vi "correlation_subVI.vi"(0 "signal":dbl[](array[numeric]), 1 "compare":dbl[](array[numeric])) -> (3 "max index":i32, 4 "max value":dbl, 5 "correlation":cluster{i32, i32, dbl[]}(graph))   [LabVIEW 2014]
uses:
  <vilib>/Analysis/2dsp.llb/1D Cross Correlation (DBL).vi
  <vilib>/Analysis/NI_AALPro.lvlib
panel:
  in  "stop":bool
  out "compare_size":i32
  out "signal_size":i32
  out "byCorrelationVI":cluster{i32, i32, "Rxy":dbl[]}(graph)
  out "compare_graph":dbl[](graph)
  out "signal_graph":dbl[](graph)
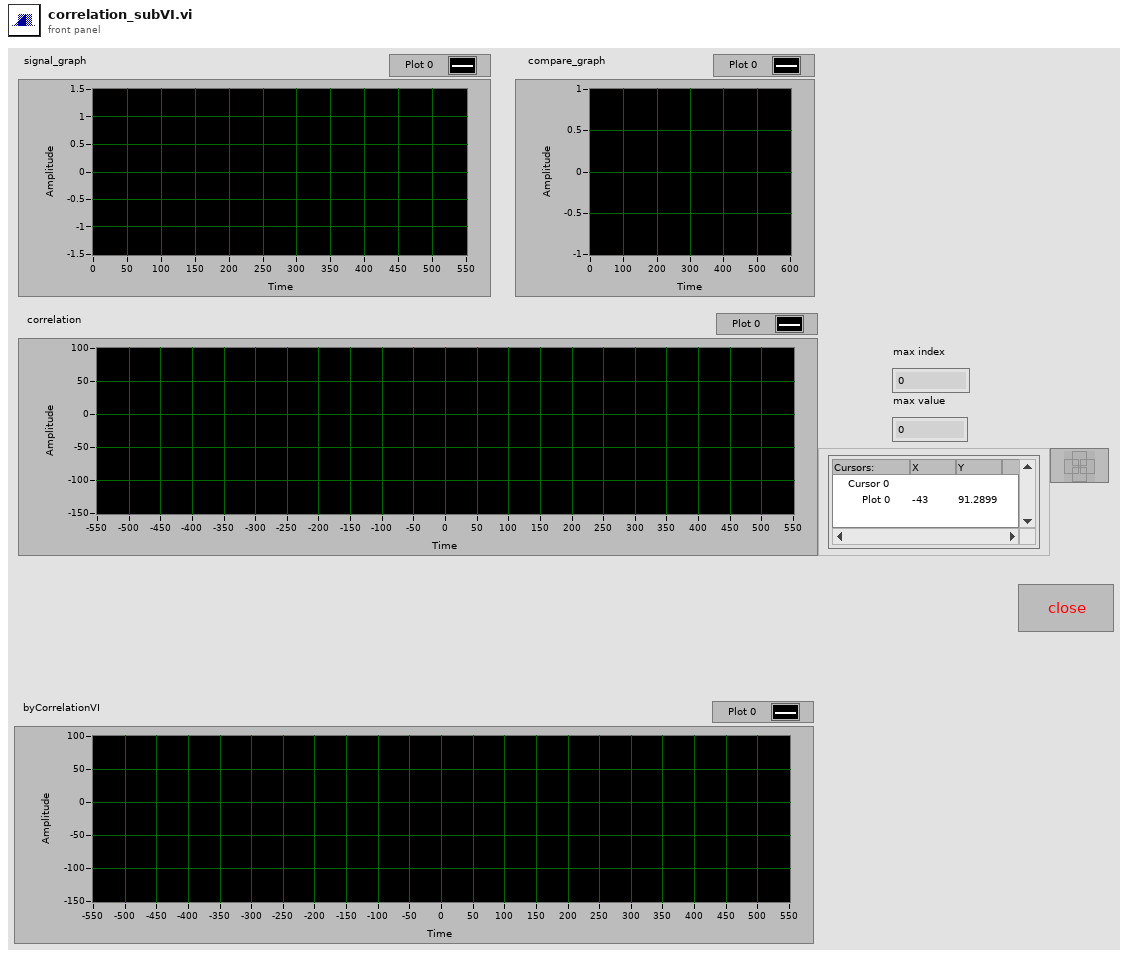
[diagram p1: front panel]
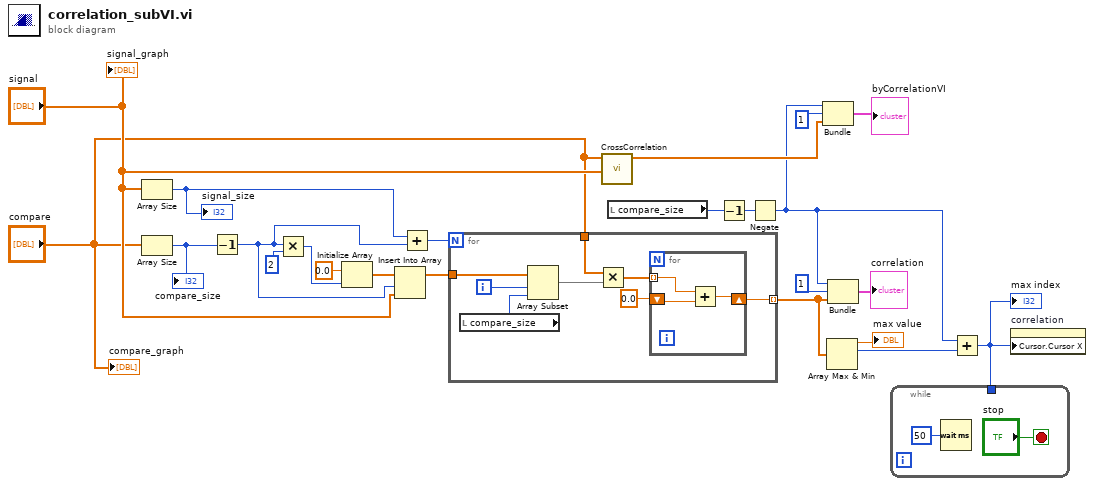
[diagram p0: block diagram]
diagram:
  n1 = Array Size(array="signal") -> (size(s)=w6:i32)
  "signal_size" <- w6
  n2 = Array Size(array="compare") -> (size(s)=w7:i32)
  "compare_size" <- w7
  n3 = Decrement(x=w7) -> (x-1=w3:i32)
  n4 = Multiply(x=w3, y=2) -> (x*y=w19:i32)
  n5 = Initialize Array(0.0 ("element"), w19) -> (w18:dbl[])
  n6 = Insert Into Array(array=w18, index=w3, new element="signal") -> (w17:dbl[])
  n7 = Add(x=w6, y=w3) -> (x+y=w22:i32)
  n8 = for {
    N: w22 -> [_]
    tunnel: [w24] -> w13 mode=indexing
    tunnel: "compare" -> [w27]
    tunnel: w17 -> [w26]
    i -> [w30]
    n9 = local read "compare_size"() -> (w25:i32)
    n10 = Array Subset(array=w26, index=w30, length=w25) -> (w28:dbl[])
    n11 = Multiply(x=w27, y=w28) -> (x*y=w31:dbl[])
    n12 = for {
      tunnel: w31 -> [w34] mode=indexing
      shift-right: [w33] -> w24
      shift-left: 0.0 -> [w32]
      n13 = Add(x=w34, y=w32) -> (x+y=w33:dbl)
    }
  }
  n14 = call-poly <vilib>:"CrossCorrelation.vi"("Y"="signal", "X"="compare") -> ("Rxy"=w11:dbl[])  [unwired: 8 in, 1 out]
  n15 = local read "compare_size"() -> (w5:i32)
  n16 = Decrement(x=w5) -> (x-1=w4:i32)
  n17 = Negate(x=w4) -> (-x=w10:i32)
  n18 = Bundle(w10, 1, "Rxy"=w11) -> (→"byCorrelationVI":cluster{i32, i32, "Rxy":dbl[]})  [unwired: 1 in]
  n19 = Array Max & Min(array=w13) -> (max value=→"max value":dbl, max index (indices)=w15:i32)  [unwired: 2 out]
  n20 = Bundle(w10, 1, w13) -> (→"correlation":cluster{i32, i32, dbl[]})  [unwired: 1 in]
  n21 = Add(x=w10, y=w15) -> (x+y=w12:i32)
  "max index" <- w12
  n22 = while {
    tunnel: w12 -> [_]
    stop <- "stop" stop-if-true
    n23 = Wait (ms)(milliseconds to wait=u32 50) -> ()  [unwired: 1 out]
  }
  n24 = property on="correlation" class="WFGraph (strict)"("Cursor.Cursor X"=w12) -> ()  [unwired: 2 in, 2 out]
  "signal_graph" <- "signal"
  "compare_graph" <- "compare"
